vi "LEP_RV_IncBuild_Clear.vi"(8 "error in (no error)":errorcluster) -> (0 "error out":errorcluster)   [LabVIEW 2011]
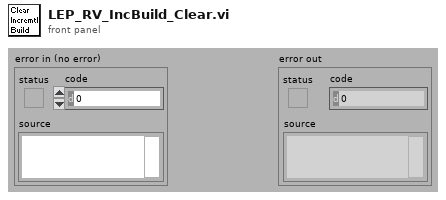
[diagram p1: front panel]
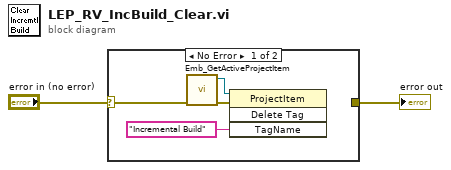
[diagram p0: block diagram]
diagram:
  n1 = case shown="No Error" "error in (no error)" {
    selector: "error in (no error)" -> [w3 w7]
    tunnel: [_ w7] -> w2
    frame No Error {
      n2 = call "Emb_GetActiveProjectItem.vi"("error in (no error)"=w3) -> ("error out"=w5:errorcluster, "ProjectItem Refnum"=w6:refnum<vi>)  [unwired: 9 out]
      n3 = invoke class="ProjectItem" method="Delete Tag"(reference=w6, error in=w5, "TagName"="Incremental Build" ("ItemName")) -> ()  [unwired: 1 in, 4 out]
    }
    frame Error {
    }
  }
  "error out" <- w2
